vi "ProcessManager.vi"() -> ()   [LabVIEW 2018]
panel:
  in  "x":i32
  in  "Play/Pause":bool
  in  "JOBS":i32=20
  out "NEW":string[](array[string])
  out "I/O WAITING":string[](array[string])
  out "RUNNING":string
  out "PRINT":string
  out "TERMINATED":string[](array[string])
  out "READY":string[](array[string])
  in  "?":bool
  out "Finished Job Table":string[][](table)
  in  "Delay (s)":i32(slide) scale=0.0..8.0
  in  "Average Printing Time":i32(slide) scale=10.0..80.0
  in  "Print Probability":i32(slide) scale=0.0..100.0
  in  "Average Process Time":i32(slide) scale=5.0..100.0
  in  "Quantum":i32(slide) scale=0.0..20.0
  in  "Probability of Job":i32(slide) scale=0.0..100.0
  out "Tiempo imprimiendo":i32
  out "quantum":i32
  out "Program Control Block":string[][](table)
  out "CLOCK":i32
  # "PROCESS MANAGER"
  # "CONTROLS"
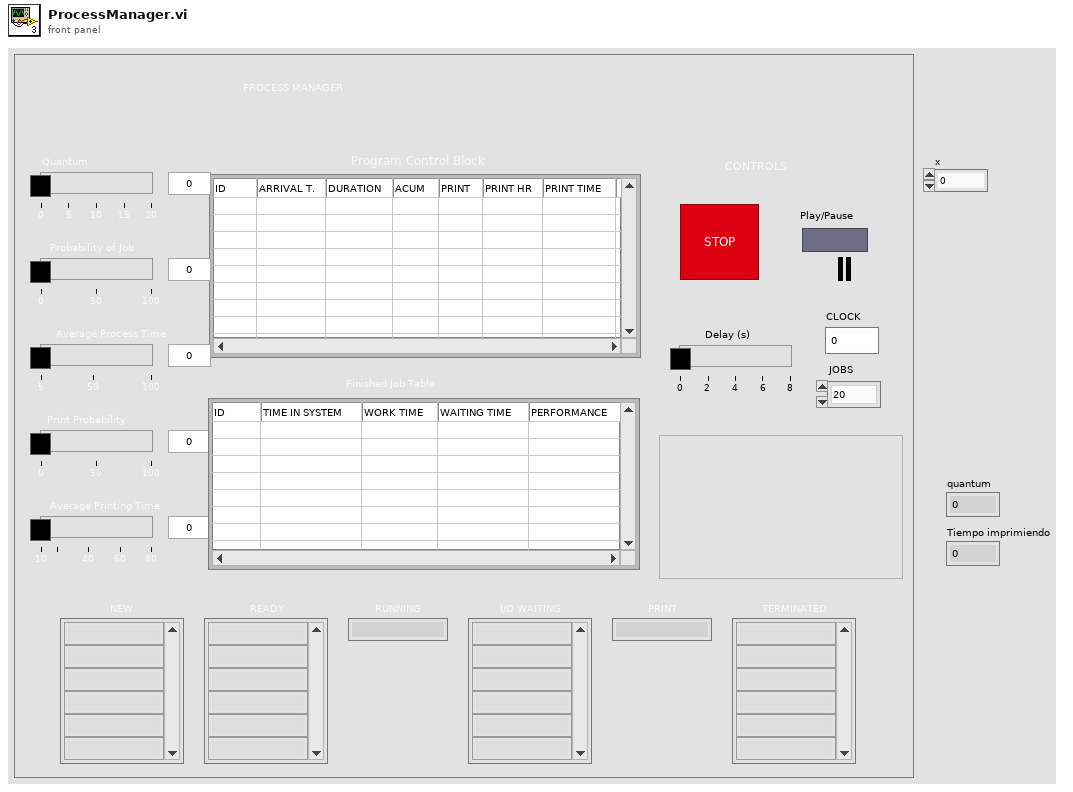
[diagram p1: front panel]
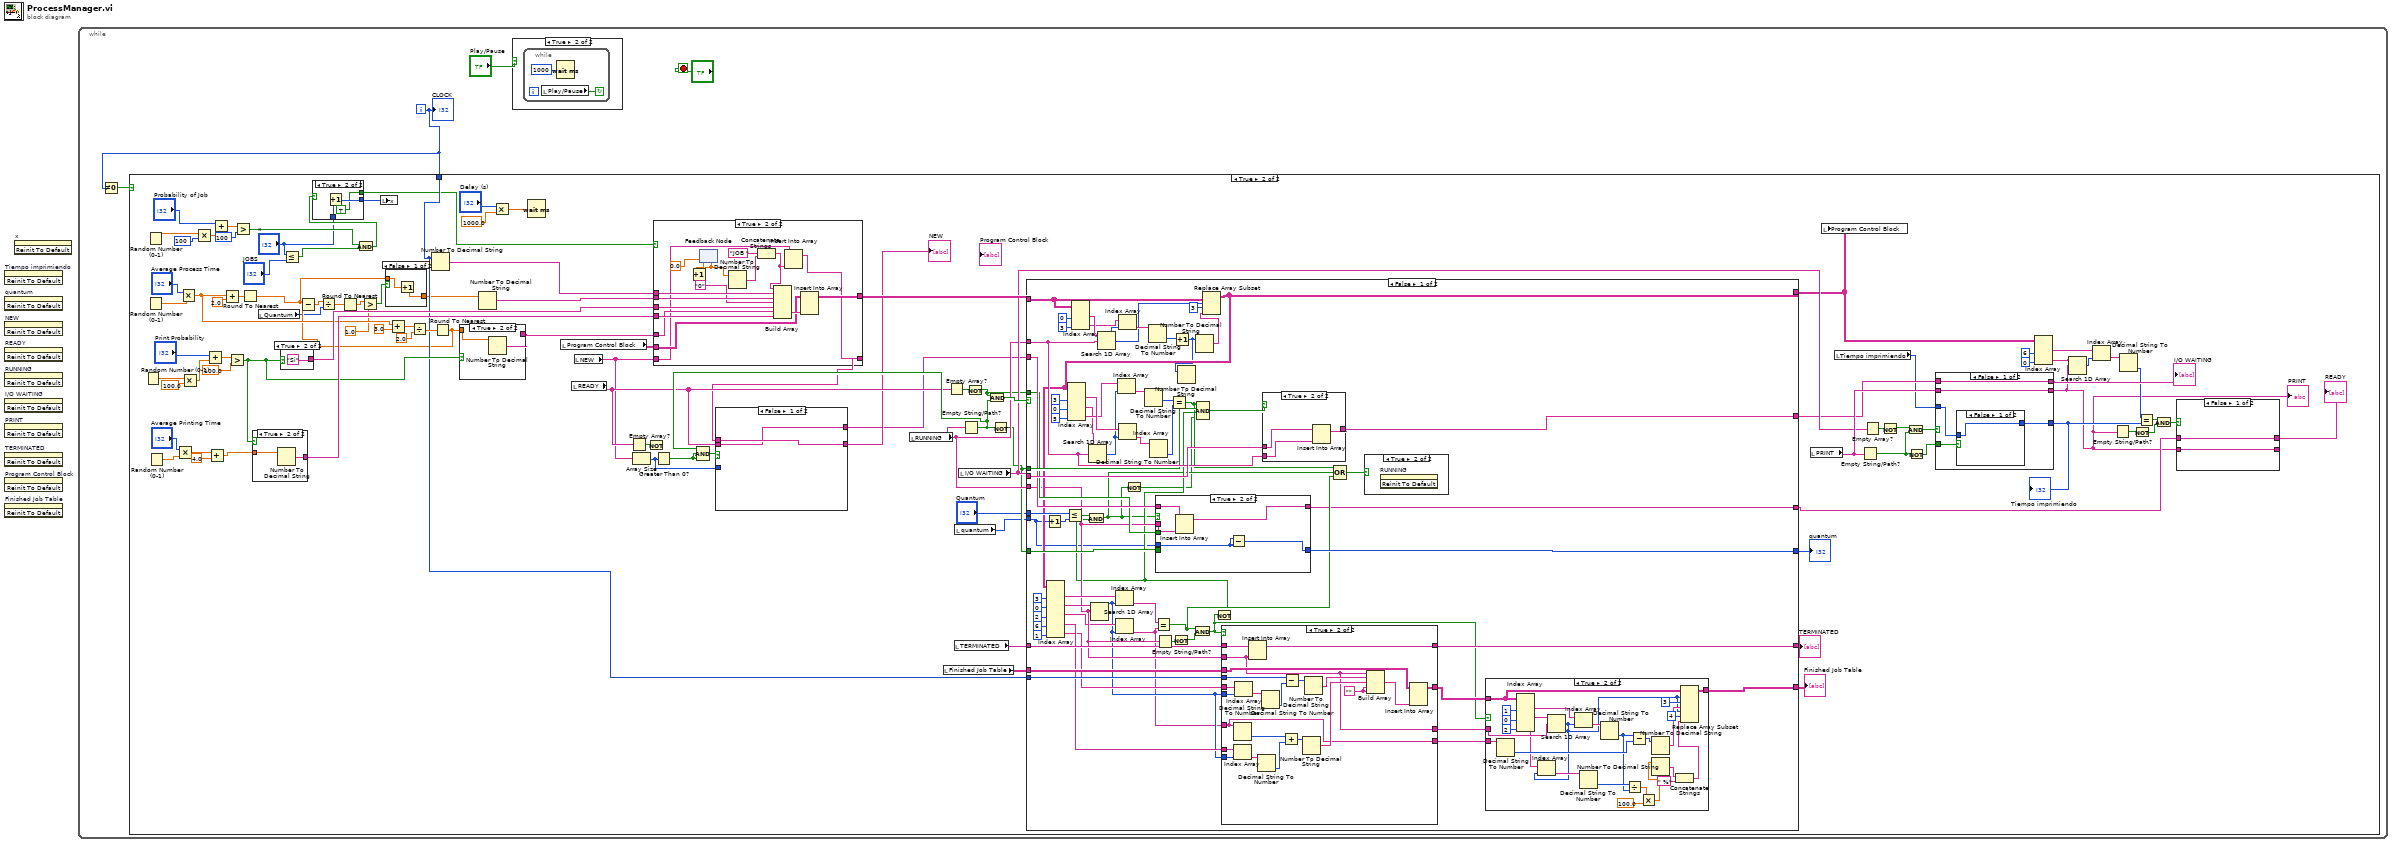
[diagram p0: block diagram]
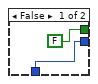
[diagram p3: hidden frame]
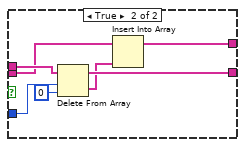
[diagram p5: hidden frame]
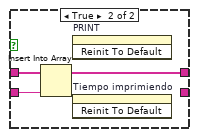
[diagram p6: hidden frame]
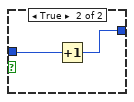
[diagram p7: hidden frame]
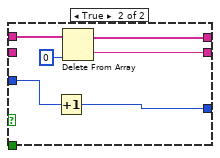
[diagram p8: hidden frame]
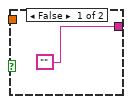
[diagram p9: hidden frame]
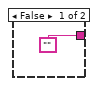
[diagram p10: hidden frame]
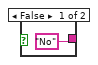
[diagram p12: hidden frame]
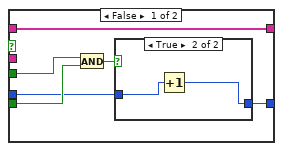
[diagram p15: hidden frame]
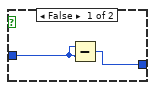
[diagram p16: hidden frame]
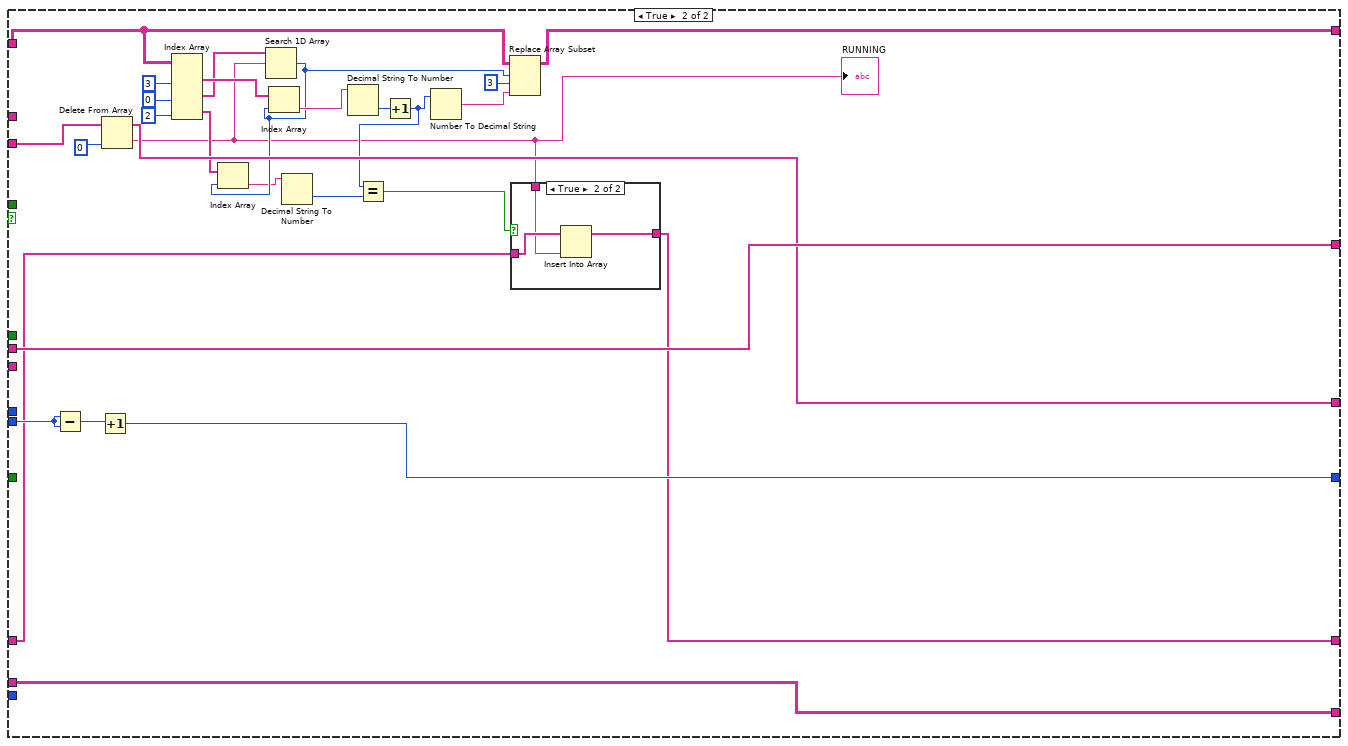
[diagram p19: hidden frame]
diagram:
  n1 = invoke on="Tiempo imprimiendo" class="DigNum (strict)" method="Reinit To Default"() -> ()  [unwired: 3 in, 3 out]
  n2 = invoke on="quantum" class="DigNum (strict)" method="Reinit To Default"() -> ()  [unwired: 3 in, 3 out]
  n3 = invoke on="NEW" class="Arr (strict)" method="Reinit To Default"() -> ()  [unwired: 3 in, 3 out]
  n4 = invoke on="READY" class="Arr (strict)" method="Reinit To Default"() -> ()  [unwired: 3 in, 3 out]
  n5 = invoke on="RUNNING" class="Str" method="Reinit To Default"() -> ()  [unwired: 3 in, 3 out]
  n6 = invoke on="I/O WAITING" class="Arr (strict)" method="Reinit To Default"() -> ()  [unwired: 3 in, 3 out]
  n7 = invoke on="PRINT" class="Str" method="Reinit To Default"() -> ()  [unwired: 3 in, 3 out]
  n8 = invoke on="TERMINATED" class="Arr (strict)" method="Reinit To Default"() -> ()  [unwired: 3 in, 3 out]
  n9 = invoke on="Program Control Block" class="Tbl (strict)" method="Reinit To Default"() -> ()  [unwired: 3 in, 3 out]
  n10 = invoke on="Finished Job Table" class="Tbl (strict)" method="Reinit To Default"() -> ()  [unwired: 3 in, 3 out]
  n11 = invoke on="x" class="DigNum (strict)" method="Reinit To Default"() -> ()  [unwired: 3 in, 3 out]
  n12 = while {
    i -> [w1]
    stop <- "?" stop-if-true
    n13 = Not Equal To 0?(x=w1) -> (x != 0?=w2:bool)
    n14 = case shown="True" w2 {
      tunnel: w1 -> [_ w33]
      frame False {
      }
      frame True {
        n15 = Random Number (0-1)() -> (number: 0 to 1=w92:dbl)
        n16 = Random Number (0-1)() -> (number: 0 to 1=w95:dbl)
        n17 = Random Number (0-1)() -> (number: 0 to 1=w98:dbl)
        n18 = Random Number (0-1)() -> (number: 0 to 1=w97:dbl)
        n19 = Multiply(x="Average Printing Time", y=w97) -> (x*y=w37:dbl)
        n20 = Multiply(x="Average Process Time", y=w98) -> (x*y=w45:dbl)
        n21 = Multiply(x=w92, y=100.0) -> (x*y=w90:dbl)
        n22 = Multiply(x=w95, y=100) -> (x*y=w93:dbl)
        n23 = Add(x="Print Probability", y=w90) -> (x+y=w105:dbl)
        n24 = Add(x=w37, y=4.0) -> (x+y=w36:dbl)
        n25 = Add(x="Probability of Job", y=w93) -> (x+y=w12:dbl)
        n26 = Add(x=w45, y=2.0) -> (x+y=w47:dbl)
        n27 = Greater?(x=w105, y=100.0) -> (0:w84:bool)
        n28 = Greater?(x=w12, y=100) -> (0:w9:bool)
        n29 = Round To Nearest(number=w47) -> (nearest integer value=w15:dbl)
        n30 = case shown="True" w84 {
          tunnel: w36 -> [_ w148]
          tunnel: ["" w147] -> w96
          frame False {
          }
          frame True {
            n31 = Number To Decimal String(number=w148) -> (decimal integer string=w147:string)  [unwired: 1 in]
          }
        }
        n32 = local read "Quantum"() -> (w21:i32)
        n33 = case shown="True" w84 {
          tunnel: ["No" "Si"] -> w99
          frame False {
          }
          frame True {
          }
        }
        n34 = Less Or Equal?(x="x", y="JOBS") -> (x <= y?=w10:bool)
        n35 = And(x=w9, y=w10) -> (x .and. y?=w8:bool)
        n36 = case shown="True" w8 {
          tunnel: "x" -> [w108 w111]
          tunnel: [w108 w110] -> w6
          tunnel: [FALSE TRUE] -> w5
          frame False {
          }
          frame True {
            n37 = Increment(x=w111) -> (x+1=w110:i32)
          }
        }
        n38 = local write "x"(w6) -> ()
        n39 = Add(x=w45, y=3.0 ("x+y")) -> (x+y=w87:dbl)
        n40 = Divide(x=w87, y=2.0) -> (x/y=w85:dbl)
        n41 = Number To Decimal String(number=w33) -> (decimal integer string=w101:string)  [unwired: 1 in]
        n42 = Round To Nearest(number=w85) -> (nearest integer value=w22:dbl)
        n43 = Subtract(x=w15, y=w22) -> (x-y=w20:dbl)
        n44 = Divide(x=w20, y=w21) -> (x/y=w19:dbl)
        n45 = Round To Nearest(number=w19) -> (nearest integer value=w18:dbl)
        n46 = Greater?(x=w18, y=1.0) -> (0:w16:bool)
        n47 = case shown="False" w16 {
          tunnel: w15 -> [w112 w114]
          tunnel: [w113 w114] -> w14
          frame False {
            n48 = Increment(x=w112) -> (x+1=w113:dbl)
          }
          frame True {
          }
        }
        n49 = case shown="True" w84 {
          tunnel: ["" w145] -> w88
          tunnel: w22 -> [_ w144]
          frame False {
          }
          frame True {
            n50 = Number To Decimal String(number=w144) -> (decimal integer string=w145:string)  [unwired: 1 in]
          }
        }
        n51 = Number To Decimal String(number=w14) -> (decimal integer string=w100:string)  [unwired: 1 in]
        n52 = Multiply(x="Delay (s)", y=1000.0 ("x*y")) -> (x*y=w102:dbl)
        n53 = Wait (ms)(milliseconds to wait=w102) -> ()  [unwired: 1 out]
        n54 = local read "Program Control Block"() -> (w82:string[][])
        n55 = local read "READY"() -> (w28:string[])
        n56 = local read "NEW"() -> (w24:string[])
        n57 = Empty Array?(array=w28) -> (empty?=w30:bool)
        n58 = Array Size(array=w24) -> (size(s)=w27:i32)
        n59 = Not(x=w30) -> ()  [unwired: 1 out]
        n60 = case shown="True" w5 {
          tunnel: w101 -> [_ w162]
          tunnel: w100 -> [_ w161]
          tunnel: [w149 w166] -> w81
          tunnel: w99 -> [_ w159]
          tunnel: w96 -> [_ w158]
          tunnel: w88 -> [_ w157]
          tunnel: w82 -> [w149 w156]
          tunnel: w24 -> [w150 w153]
          tunnel: [w150 w152] -> w13
          frame False {
          }
          frame True {
            n61 = feedback #1(0.0) -> (w163:dbl)
            n62 = Increment(x=w163) -> (x+1=w164:dbl)
            n63 = feedback-in #1(w164) -> ()
            n64 = Number To Decimal String(number=w163) -> (decimal integer string=w155:string)  [unwired: 1 in]
            n65 = Concatenate Strings("JOB ", w155) -> (w154:string)
            n66 = Build Array(w154, w162, w161, "0", w159, w157, w158) -> (w167:string[])
            n67 = Insert Into Array(array=w153, new element=w154) -> (w152:string[])  [unwired: 1 in]
            n68 = Insert Into Array(array=w156, new element=w167) -> (w166:string[][])  [unwired: 2 in]
          }
        }
        n69 = Greater Than 0?(x=w27) -> (x > 0?=w23:bool)
        n70 = local read "RUNNING"() -> (w73:string)
        n71 = local read "Finished Job Table"() -> (w34:string[][])
        n72 = Empty Array?(array=w28) -> (empty?=w89:bool)
        n73 = local read "TERMINATED"() -> (w49:string[])
        n74 = local read "quantum"() -> (w69:i32)
        n75 = local read "I/O WAITING"() -> (w76:string[])
        n76 = Empty String/Path?(string/path=w73) -> (empty?=w29:bool)
        n77 = Compound Arithmetic op=AND(w29, w23, w23) -> (w31:bool)
        n78 = case shown="False" w31 {
          tunnel: w28 -> [w115 w119]
          tunnel: w13 -> [w116 w123]
          tunnel: w27 -> [_ w122]
          tunnel: [w116 w121] -> w26
          tunnel: [w115 w118] -> w25
          frame False {
          }
          frame True {
            n79 = Delete From Array(array=w123, length=w122, index=0) -> (deleted portion=w120:string[], array with subset deleted=w121:string[])
            n80 = Insert Into Array(array=w119, new element=w120) -> (w118:string[])  [unwired: 1 in]
          }
        }
        "NEW" <- w26
        n81 = Not(x=w89) -> (.not. x?=w71:bool)
        n82 = And(x=w71, y=w29) -> (x .and. y?=w83:bool)
        n83 = Not(x=w29) -> (.not. x?=w72:bool)
        n84 = case shown="False" w83 {
          tunnel: w25 -> [w213 w336]
          tunnel: w73 -> [w219 _]
          tunnel: w81 -> [w197 w327]
          tunnel: [w196 w326] -> w67
          tunnel: w76 -> [w220 w325]
          tunnel: [w218 w325] -> w75
          tunnel: w72 -> [w214 _]
          tunnel: [w170 w324] -> w51
          tunnel: w73 -> [w191 _]
          tunnel: w69 -> [w175 w323]
          tunnel: "Quantum" -> [w211 _]
          tunnel: [w208 w321] -> w70
          tunnel: w72 -> [w212 _]
          tunnel: w71 -> [w210 _]
          tunnel: w49 -> [w202 w313]
          tunnel: [w201 w311] -> w48
          tunnel: w34 -> [w194 w310]
          tunnel: w33 -> [w193 _]
          tunnel: [w189 w310] -> w32
          frame False {
            n85 = Increment(x=w175) -> (x+1=w176:i32)
            n86 = Less Or Equal?(x=w211, y=w176) -> (x <= y?=w195:bool)
            n87 = Index Array(array=w197, index (col) #1=0 ("disabled index (col)"), index (col) #2=3 ("index (col)")) -> (element #1=w235:string[], element #2=w234:string[])  [unwired: 2 in]
            n88 = Search 1D Array(1D array=w235, element=w219) -> (index of element=w231:i32)  [unwired: 1 in]
            n89 = Index Array(array=w234, index=w231) -> (element=w233:string)
            n90 = Decimal String To Number(string=w233) -> (number=w174:i32)  [unwired: 2 in, 1 out]
            n91 = Empty String/Path?(string/path=w191) -> (empty?=w200:bool)
            n92 = Not(x=w200) -> (.not. x?=w199:bool)
            n93 = Increment(x=w174) -> (x+1=w172:i32)
            n94 = Number To Decimal String(number=w172) -> ()  [unwired: 1 in, 1 out]
            n95 = Number To Decimal String(number=w172) -> (decimal integer string=w230:string)  [unwired: 1 in]
            n96 = Replace Array Subset(array=w197, new element=w230, index (row)=w231, index (col)=3 ("disabled index (col)")) -> (w196:string[][])
            n97 = Index Array(array=w196, index (col) #1=3 ("disabled index (col)"), index (col) #2=0 ("index (col)"), index (col) #3=2 ("index (col)"), index (col) #4=6 ("index (col)"), index (col) #5=1 ("index (col)")) -> (element #1=w204:string[], element #2=w205:string[], element #3=w187:string[], element #4=w186:string[], element #5=w184:string[])  [unwired: 5 in]
            n98 = Index Array(array=w196, index (col) #1=3 ("disabled index (col)"), index (col) #2=0 ("disabled index (col)"), index (col) #3=5 ("index (col)")) -> (element #1=w227:string[], element #2=w216:string[], element #3=w217:string[])  [unwired: 3 in]
            n99 = Search 1D Array(1D array=w216, element=w219) -> (index of element=w223:i32)  [unwired: 1 in]
            n100 = Search 1D Array(1D array=w205, element=w191) -> (index of element=w177:i32)  [unwired: 1 in]
            n101 = Index Array(array=w187, index=w177) -> (element=w173:string)
            n102 = Index Array(array=w204, index=w177) -> (element=w171:string)
            n103 = Index Array(array=w217, index=w223) -> (element=w222:string)
            n104 = Index Array(array=w227, index=w223) -> (element=w226:string)
            n105 = Decimal String To Number(string=w222) -> (number=w221:i32)  [unwired: 2 in, 1 out]
            n106 = Decimal String To Number(string=w226) -> (number=w225:i32)  [unwired: 2 in, 1 out]
            n107 = Equal?(x=w171, y=w173) -> (x = y?=w198:bool)
            n108 = Equal?(x=w221, y=w225) -> (x = y?=w209:bool)
            n109 = Compound Arithmetic op=AND(w198, w199) -> (w178:bool)
            n110 = Not(x=w178) -> (.not. x?=w181:bool)
            n111 = Compound Arithmetic op=AND(w195, w181) -> (w180:bool)
            n112 = Not(x=w180) -> (.not. x?=w179:bool)
            n113 = case shown="True" w180 {
              tunnel: w191 -> [_ w305]
              tunnel: w213 -> [w294 w304]
              tunnel: [w294 w303] -> w170
              tunnel: w210 -> [w296 _]
              tunnel: w212 -> [w293 _]
              tunnel: w175 -> [w292 w302]
              tunnel: [w291 w301] -> w208
              frame False {
                n114 = And(x=w296, y=w293) -> (x .and. y?=w295:bool)
                n115 = case shown="True" w295 {
                  tunnel: w292 -> [w298 w300]
                  tunnel: [w297 w299] -> w291
                  frame False {
                    n116 = Subtract(x=w298, y=w298) -> (x-y=w297:i32)
                  }
                  frame True {
                    n117 = Increment(x=w300) -> (x+1=w299:i32)
                  }
                }
              }
              frame True {
                n118 = Insert Into Array(array=w304, new element=w305) -> (w303:string[])  [unwired: 1 in]
                n119 = Subtract(x=w302, y=w302) -> (x-y=w301:i32)
              }
            }
            n120 = Compound Arithmetic op=AND(w209, w214, w181, w179) -> (w182:bool)
            n121 = case shown="True" w178 {
              tunnel: w202 -> [w268 w290]
              tunnel: w191 -> [w265 w269]
              tunnel: [w268 w289] -> w201
              tunnel: w194 -> [w267 w273]
              tunnel: w193 -> [_ w288]
              tunnel: w184 -> [_ w287]
              tunnel: w177 -> [_ w286]
              tunnel: w173 -> [w266 w271]
              tunnel: w186 -> [_ w280]
              tunnel: w177 -> [_ w279]
              tunnel: [w267 w274] -> w190
              tunnel: [w266 w271] -> w188
              tunnel: [w265 w269] -> w183
              frame False {
              }
              frame True {
                w270 = "" ("element")
                n122 = Index Array(array=w280, index=w279) -> (element=w278:string)
                n123 = Decimal String To Number(string=w271) -> (number=w281:i32)  [unwired: 2 in, 1 out]
                n124 = Index Array(array=w287, index=w286) -> (element=w285:string)
                n125 = Insert Into Array(array=w290, new element=w269) -> (w289:string[])  [unwired: 1 in]
                n126 = Decimal String To Number(string=w278) -> (number=w277:i32)  [unwired: 2 in, 1 out]
                n127 = Decimal String To Number(string=w285) -> (number=w284:i32)  [unwired: 2 in, 1 out]
                n128 = Add(x=w281, y=w277) -> (x+y=w276:i32)
                n129 = Subtract(x=w288, y=w284) -> (x-y=w283:i32)
                n130 = Number To Decimal String(number=w276) -> (decimal integer string=w275:string)  [unwired: 1 in]
                n131 = Number To Decimal String(number=w283) -> (decimal integer string=w282:string)  [unwired: 1 in]
                n132 = Build Array(w269, w282, w275, w270, w270) -> (w272:string[])
                n133 = Insert Into Array(array=w273, new element=w272) -> (w274:string[][])  [unwired: 2 in]
              }
            }
            n134 = case shown="True" w182 {
              tunnel: w220 -> [w306 w309]
              tunnel: w219 -> [_ w308]
              tunnel: [w306 w307] -> w218
              frame False {
              }
              frame True {
                n135 = Insert Into Array(array=w309, new element=w308) -> (w307:string[])  [unwired: 1 in]
              }
            }
            n136 = Compound Arithmetic op=OR(w209, w180, w198) -> (w215:bool)
            n137 = case shown="True" w215 {
              frame False {
              }
              frame True {
                n138 = invoke on="RUNNING" class="Str" method="Reinit To Default"() -> ()  [unwired: 3 in, 3 out]
              }
            }
            n139 = case shown="True" w178 {
              tunnel: w190 -> [w238 w263]
              tunnel: [w238 w252] -> w189
              tunnel: w188 -> [_ w264]
              tunnel: w183 -> [_ w261]
              frame False {
              }
              frame True {
                n140 = Decimal String To Number(string=w264) -> (number=w256:i32)  [unwired: 2 in, 1 out]
                n141 = Index Array(array=w263, index (col) #1=1 ("disabled index (col)"), index (col) #2=0 ("index (col)"), index (col) #3=2 ("index (col)")) -> (element #1=w258:string[], element #2=w259:string[], element #3=w250:string[])  [unwired: 3 in]
                n142 = Search 1D Array(1D array=w259, element=w261) -> (index of element=w245:i32)  [unwired: 1 in]
                n143 = Index Array(array=w250, index=w245) -> (element=w249:string)
                n144 = Index Array(array=w258, index=w245) -> (element=w257:string)
                n145 = Decimal String To Number(string=w249) -> (number=w248:i32)  [unwired: 2 in, 1 out]
                n146 = Decimal String To Number(string=w257) -> (number=w247:i32)  [unwired: 2 in, 1 out]
                n147 = Divide(x=w248, y=w247) -> (x/y=w244:dbl)
                n148 = Subtract(x=w247, y=w256) -> (x-y=w255:i32)
                n149 = Multiply(x=w244, y=100.0) -> (x*y=w242:dbl)
                n150 = Number To Decimal String(number=w255) -> (decimal integer string=w254:string)  [unwired: 1 in]
                n151 = Number To Decimal String(number=w242) -> (decimal integer string=w241:string)  [unwired: 1 in]
                n152 = Concatenate Strings(w241, " %" ("string")) -> (w239:string)
                n153 = Replace Array Subset(array=w263, new element #1=w254, index (row) #1=w245, index (col) #1=3 ("disabled index (col)"), new element #2=w239, index (row) #2=w245, index (col) #2=4 ("index (col)")) -> (w252:string[][])
              }
            }
          }
          frame True {
            n154 = Subtract(x=w323, y=w323) -> (x-y=w322:i32)
            n155 = Increment(x=w322) -> (x+1=w321:i32)
            n156 = Delete From Array(array=w336, index=0) -> (deleted portion=w312:string, array with subset deleted=w324:string[])  [unwired: 1 in]
            "RUNNING" <- w312
            n157 = Index Array(array=w327, index (col) #1=3 ("disabled index (col)"), index (col) #2=0 ("index (col)"), index (col) #3=2 ("index (col)")) -> (element #1=w333:string[], element #2=w332:string[], element #3=w319:string[])  [unwired: 3 in]
            n158 = Search 1D Array(1D array=w332, element=w312) -> (index of element=w318:i32)  [unwired: 1 in]
            n159 = Index Array(array=w319, index=w318) -> (element=w317:string)
            n160 = Index Array(array=w333, index=w318) -> (element=w331:string)
            n161 = Decimal String To Number(string=w317) -> (number=w315:i32)  [unwired: 2 in, 1 out]
            n162 = Decimal String To Number(string=w331) -> (number=w330:i32)  [unwired: 2 in, 1 out]
            n163 = Increment(x=w330) -> (x+1=w316:i32)
            n164 = Equal?(x=w316, y=w315) -> (x = y?=w314:bool)
            n165 = Number To Decimal String(number=w316) -> (decimal integer string=w328:string)  [unwired: 1 in]
            n166 = Replace Array Subset(array=w327, new element=w328, index (row)=w318, index (col)=3 ("disabled index (col)")) -> (w326:string[][])
            n167 = case shown="True" w314 {
              tunnel: w313 -> [w338 w341]
              tunnel: w312 -> [_ w340]
              tunnel: [w338 w339] -> w311
              frame False {
              }
              frame True {
                n168 = Insert Into Array(array=w341, new element=w340) -> (w339:string[])  [unwired: 1 in]
              }
            }
          }
        }
        "quantum" <- w70
        "TERMINATED" <- w48
        "Finished Job Table" <- w32
        n169 = local read "PRINT"() -> (w77:string)
        n170 = local write "Program Control Block"(w67) -> ()
        n171 = local read "Tiempo imprimiendo"() -> (w68:i32)
        n172 = Empty String/Path?(string/path=w77) -> (empty?=w57:bool)
        n173 = Empty Array?(array=w76) -> (empty?=w79:bool)
        n174 = Not(x=w79) -> (.not. x?=w78:bool)
        n175 = And(x=w78, y=w57) -> (x .and. y?=w58:bool)
        n176 = Not(x=w57) -> (.not. x?=w56:bool)
        n177 = case shown="False" w58 {
          tunnel: w75 -> [w132 w142]
          tunnel: [w133 w141] -> w38
          tunnel: w77 -> [w133 _]
          tunnel: [w132 w140] -> w74
          tunnel: w68 -> [w130 w138]
          tunnel: [w129 w137] -> w59
          tunnel: w56 -> [w131 _]
          frame False {
            n178 = case shown="False" w131 {
              tunnel: w130 -> [w134 w136]
              tunnel: [w134 w135] -> w129
              frame False {
              }
              frame True {
                n179 = Increment(x=w136) -> (x+1=w135:i32)
              }
            }
          }
          frame True {
            n180 = Increment(x=w138) -> (x+1=w137:i32)
            n181 = Delete From Array(array=w142, index=0) -> (deleted portion=w141:string, array with subset deleted=w140:string[])  [unwired: 1 in]
          }
        }
        "I/O WAITING" <- w74
        "PRINT" <- w38
        "Tiempo imprimiendo" <- w59
        n182 = Index Array(array=w67, index (col) #1=6 ("disabled index (col)"), index (col) #2=0 ("index (col)")) -> (element #1=w62:string[], element #2=w64:string[])  [unwired: 2 in]
        n183 = Search 1D Array(1D array=w64, element=w38) -> (index of element=w63:i32)  [unwired: 1 in]
        n184 = Index Array(array=w62, index=w63) -> (element=w61:string)
        n185 = Empty String/Path?(string/path=w38) -> (empty?=w55:bool)
        n186 = Decimal String To Number(string=w61) -> (number=w60:i32)  [unwired: 2 in, 1 out]
        n187 = Not(x=w55) -> (.not. x?=w52:bool)
        n188 = Equal?(x=w60, y=w59) -> (x = y?=w54:bool)
        n189 = And(x=w54, y=w52) -> (x .and. y?=w53:bool)
        n190 = case shown="False" w53 {
          tunnel: w51 -> [w125 w128]
          tunnel: w38 -> [w124 w127]
          tunnel: [w125 w126] -> w50
          tunnel: [w124 _] -> _
          frame False {
          }
          frame True {
            n191 = Insert Into Array(array=w128, new element=w127) -> (w126:string[])  [unwired: 1 in]
            n192 = invoke on="PRINT" class="Str" method="Reinit To Default"() -> ()  [unwired: 3 in, 3 out]
            n193 = invoke on="Tiempo imprimiendo" class="DigNum (strict)" method="Reinit To Default"() -> ()  [unwired: 3 in, 3 out]
          }
        }
        "READY" <- w50
      }
    }
    n194 = case shown="True" "Play/Pause" {
      frame False {
      }
      frame True {
        n195 = while {
          stop <- w342 continue-if-true
          n196 = local read "Play/Pause"() -> (w342:bool)
          n197 = Wait (ms)(milliseconds to wait=u32 1000) -> ()  [unwired: 1 out]
        }
      }
    }
    "CLOCK" <- w1
  }
